vi "parse.vi"(8 "error in (no error)":errorcluster, 10 "DynamicFrameParser":refnum<class "DynamicFrameParser.lvclass">, 11 "ILC in":refnum<class "ILC.lvclass">) -> (0 "error out":errorcluster, 2 "ParseSuccessful":bool, 3 "ILC out":refnum<class "ILC.lvclass">)   [LabVIEW 2015, in "RTILC.lvlib" / "ILC.lvclass"]
uses:
  ILC.lvclass
  Common_RT_Modbus/DynamicFrameParser/DynamicFrameParser.lvclass
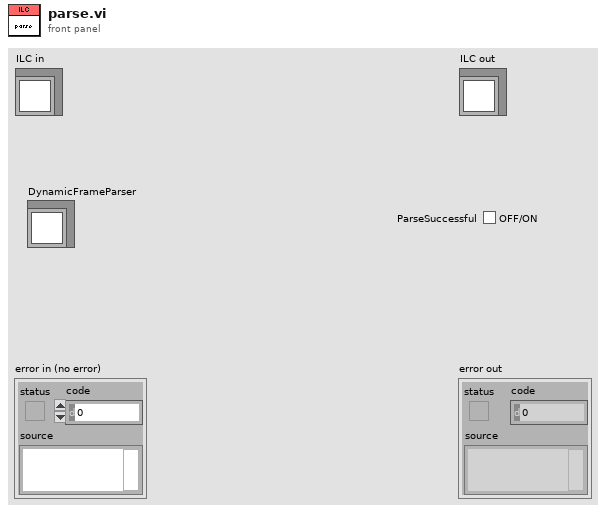
[diagram p1: front panel]
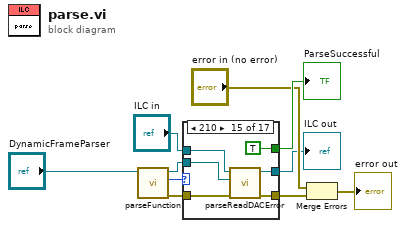
[diagram p0: block diagram]
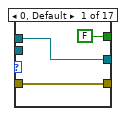
[diagram p2: hidden frame]
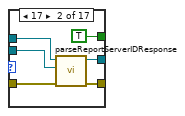
[diagram p3: hidden frame]
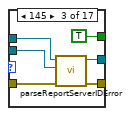
[diagram p4: hidden frame]
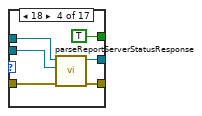
[diagram p5: hidden frame]
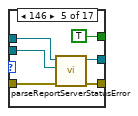
[diagram p6: hidden frame]
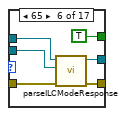
[diagram p7: hidden frame]
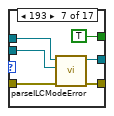
[diagram p8: hidden frame]
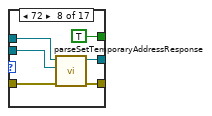
[diagram p9: hidden frame]
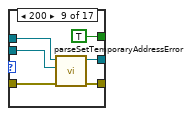
[diagram p10: hidden frame]
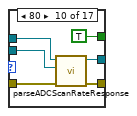
[diagram p11: hidden frame]
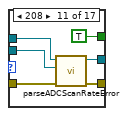
[diagram p12: hidden frame]
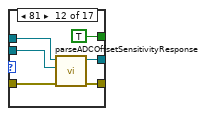
[diagram p13: hidden frame]
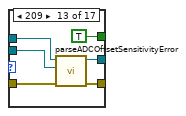
[diagram p14: hidden frame]
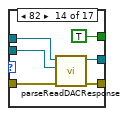
[diagram p15: hidden frame]
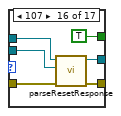
[diagram p16: hidden frame]
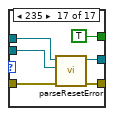
[diagram p17: hidden frame]
diagram:
  n1 = call "parseFunction.vi"("FrameParser in"="DynamicFrameParser") -> ("error out"=w6:errorcluster, "Function"=w9:u8, "FrameParser out"=w2:refnum<class "DynamicFrameParser.lvclass">)  [unwired: 8 in]
  n2 = case shown="210" w9 {
    tunnel: [FALSE TRUE TRUE TRUE TRUE TRUE TRUE TRUE TRUE TRUE TRUE TRUE TRUE TRUE TRUE TRUE TRUE] -> w8
    tunnel: w6 -> [w12 w17 w23 w28 w34 w41 w47 w53 w59 w65 w71 w77 w83 w89 w95 w101 w107]
    tunnel: [w12 w16 w22 w27 w33 w40 w46 w52 w58 w64 w70 w76 w82 w88 w94 w100 w106] -> w5
    tunnel: "ILC in" -> [w11 w19 w25 w31 w37 w42 w49 w55 w61 w67 w73 w79 w85 w91 w97 w103 w109]
    tunnel: w2 -> [_ w18 w24 w29 w35 w43 w48 w54 w60 w66 w72 w78 w84 w90 w96 w102 w108]
    tunnel: [w11 w15 w21 w30 w36 w39 w45 w51 w57 w63 w69 w75 w81 w87 w93 w99 w105] -> w1
    frame 0, Default {
    }
    frame 17 {
      n3 = call "parseReportServerIDResponse.vi"("error in (no error)"=w17, "DynamicFrameParser"=w18, "ILC in"=w19) -> ("error out"=w16:errorcluster, "ILC out"=w15:refnum<class "ILC.lvclass">)  [unwired: 7 in]
    }
    frame 145 {
      n4 = call "parseReportServerIDError.vi"("error in (no error)"=w23, "DynamicFrameParser"=w24, "ILC in"=w25) -> ("error out"=w22:errorcluster, "ILC out"=w21:refnum<class "ILC.lvclass">)  [unwired: 7 in]
    }
    frame 18 {
      n5 = call "parseReportServerStatusResponse.vi"("error in (no error)"=w28, "DynamicFrameParser"=w29, "ILC in"=w31) -> ("error out"=w27:errorcluster, "ILC out"=w30:refnum<class "ILC.lvclass">)  [unwired: 7 in]
    }
    frame 146 {
      n6 = call "parseReportServerStatusError.vi"("error in (no error)"=w34, "DynamicFrameParser"=w35, "ILC in"=w37) -> ("error out"=w33:errorcluster, "ILC out"=w36:refnum<class "ILC.lvclass">)  [unwired: 7 in]
    }
    frame 65 {
      n7 = call "parseILCModeResponse.vi"("error in (no error)"=w41, "DynamicFrameParser"=w43, "ILC in"=w42) -> ("error out"=w40:errorcluster, "ILC out"=w39:refnum<class "ILC.lvclass">)  [unwired: 7 in]
    }
    frame 193 {
      n8 = call "parseILCModeError.vi"("error in (no error)"=w47, "DynamicFrameParser"=w48, "ILC in"=w49) -> ("error out"=w46:errorcluster, "ILC out"=w45:refnum<class "ILC.lvclass">)  [unwired: 7 in]
    }
    frame 72 {
      n9 = call "parseSetTemporaryAddressResponse.vi"("error in (no error)"=w53, "DynamicFrameParser"=w54, "ILC in"=w55) -> ("error out"=w52:errorcluster, "ILC out"=w51:refnum<class "ILC.lvclass">)  [unwired: 7 in]
    }
    frame 200 {
      n10 = call "parseSetTemporaryAddressError.vi"("error in (no error)"=w59, "DynamicFrameParser"=w60, "ILC in"=w61) -> ("error out"=w58:errorcluster, "ILC out"=w57:refnum<class "ILC.lvclass">)  [unwired: 7 in]
    }
    frame 80 {
      n11 = call "parseADCScanRateResponse.vi"("error in (no error)"=w65, "DynamicFrameParser"=w66, "ILC in"=w67) -> ("error out"=w64:errorcluster, "ILC out"=w63:refnum<class "ILC.lvclass">)  [unwired: 7 in]
    }
    frame 208 {
      n12 = call "parseADCScanRateError.vi"("error in (no error)"=w71, "DynamicFrameParser"=w72, "ILC in"=w73) -> ("error out"=w70:errorcluster, "ILC out"=w69:refnum<class "ILC.lvclass">)  [unwired: 7 in]
    }
    frame 81 {
      n13 = call "parseADCOffsetSensitivityResponse.vi"("error in (no error)"=w77, "DynamicFrameParser"=w78, "ILC in"=w79) -> ("error out"=w76:errorcluster, "ILC out"=w75:refnum<class "ILC.lvclass">)  [unwired: 7 in]
    }
    frame 209 {
      n14 = call "parseADCOffsetSensitivityError.vi"("error in (no error)"=w83, "DynamicFrameParser"=w84, "ILC in"=w85) -> ("error out"=w82:errorcluster, "ILC out"=w81:refnum<class "ILC.lvclass">)  [unwired: 7 in]
    }
    frame 82 {
      n15 = call "parseReadDACResponse.vi"("error in (no error)"=w89, "DynamicFrameParser"=w90, "ILC in"=w91) -> ("error out"=w88:errorcluster, "ILC out"=w87:refnum<class "ILC.lvclass">)  [unwired: 7 in]
    }
    frame 210 {
      n16 = call "parseReadDACError.vi"("error in (no error)"=w95, "DynamicFrameParser"=w96, "ILC in"=w97) -> ("error out"=w94:errorcluster, "ILC out"=w93:refnum<class "ILC.lvclass">)  [unwired: 7 in]
    }
    frame 107 {
      n17 = call "parseResetResponse.vi"("error in (no error)"=w101, "DynamicFrameParser"=w102, "ILC in"=w103) -> ("error out"=w100:errorcluster, "ILC out"=w99:refnum<class "ILC.lvclass">)  [unwired: 7 in]
    }
    frame 235 {
      n18 = call "parseResetError.vi"("error in (no error)"=w107, "DynamicFrameParser"=w108, "ILC in"=w109) -> ("error out"=w106:errorcluster, "ILC out"=w105:refnum<class "ILC.lvclass">)  [unwired: 7 in]
    }
  }
  "ILC out" <- w1
  "ParseSuccessful" <- w8
  n19 = Merge Errors("error in (no error)", w5) -> (→"error out":errorcluster)
